vi "Write DefaultAlternateCellBGKColor.vi"(8 "error in (no error)":errorcluster, 10 "CellBGKColorAlternate":u32(colorbox)=15790320, 11 "DataGridView in":refnum<class "DataGridView.lvclass">) -> (0 "error out":errorcluster, 3 "DataGridView out":refnum<class "DataGridView.lvclass">)   [LabVIEW 2016, in "DataGrid.lvlib" / "DataGridView.lvclass"]
uses:
  <userlib>/LabVIEWdotNetDataGrid/source/DataGridView/DataGridView.lvclass
  System.Drawing
  <userlib>/LabVIEWdotNetDataGrid/source/DataGridView/DataGridView.lvclass/DataGridView.ctl
  System.Windows.Forms
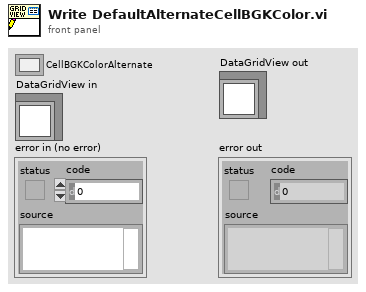
[diagram p1: front panel]
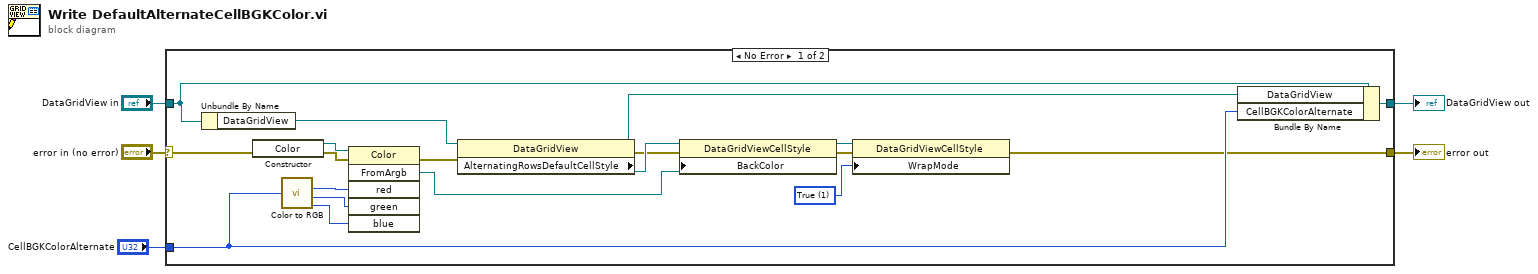
[diagram p0: block diagram]
diagram:
  n1 = case shown="No Error" "error in (no error)" {
    selector: "error in (no error)" -> [w16 w25]
    tunnel: [w7 w25] -> w4
    tunnel: [w24 w26] -> w2
    tunnel: "DataGridView in" -> [w18 w26]
    tunnel: "CellBGKColorAlternate" -> [w15 _]
    frame No Error {
      w10 = 1 items=["NotSet", "True", "False"] ("WrapMode")
      n2 = Unbundle By Name(w18) -> ("DataGridView"=w17:refnum<k24>)
      n3 = constructor class="Color"(error in=w16) -> (reference out=w19:refnum<k24>, error out=w20:errorcluster)  [unwired: 2 in, 1 out]
      n4 = call <vilib>:"Color to RGB.vi"("Color"=w15) -> ("R"=w21:u8, "G"=w22:u8, "B"=w23:u8)  [unwired: 1 out]
      n5 = invoke class="Color" method="FromArgb"(reference=w19, error in=w20, "red"=w21, "green"=w22, "blue"=w23) -> (error out=w11:errorcluster, "FromArgb"=w14:refnum<k24>)  [unwired: 1 in, 4 out]
      n6 = property class="DataGridView"(reference=w17, error in=w11) -> (reference out=w6:refnum<k24>, error out=w12:errorcluster, "AlternatingRowsDefaultCellStyle"=w13:refnum<k24>)
      n7 = property class="DataGridViewCellStyle"(reference=w13, error in=w12, "BackColor"=w14) -> (reference out=w9:refnum<k24>, error out=w8:errorcluster)
      n8 = property class="DataGridViewCellStyle"(reference=w9, error in=w8, "WrapMode"=w10) -> (error out=w7:errorcluster)  [unwired: 1 out]
      n9 = Bundle By Name(cluster=w18, "DataGridView"=w6, "CellBGKColorAlternate"=w15) -> (w24:refnum<class "DataGridView.lvclass">)
    }
    frame Error {
    }
  }
  "error out" <- w4
  "DataGridView out" <- w2
